vi "PolyVI.vi"   [LabVIEW 2017]
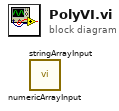
[diagram p0: block diagram]
diagram:
  n1 = call "numericArrayInput.vi"() -> ()  [unwired: 11 in, 1 out]
  n2 = call "stringArrayInput.vi"() -> ()  [unwired: 12 in]
